vi "CHS-simulate-dashboard.vi"() -> ()   [LabVIEW 2019]
uses:
  Swerve_Drive_System/CHS_DRIVE_GLOBALS.vi
  Simulation/CHS_SIM_SIM_Globals.vi
  Trajectory Following/CHS_TRAJECTORY_GLOBALS.vi
  <vilib>/Rock Robotics/WPI/ThirdParty/JAS_Junk/TrajLib/Trajectory_Library.lvlib
  Vision_Interface/CHS_Vision_Globals.vi
  <vilib>/Rock Robotics/WPI/ThirdParty/ChoreoLib/ChoreoLib.lvlib
  <vilib>/Rock Robotics/WPI/ThirdParty/JAS_Junk/TrajLib/TypeDef/ROTATION2D.ctl
  <vilib>/Rock Robotics/WPI/ThirdParty/JAS_Junk/TrajLib/TypeDef/CHASSIS_SPEEDS.ctl
  <vilib>/Rock Robotics/WPI/ThirdParty/JAS_Junk/TrajLib/TypeDef/TRANSLATION2D.ctl
  <vilib>/Rock Robotics/WPI/ThirdParty/JAS_Junk/TrajLib/TypeDef/POSE2D.ctl
panel:
  in  "Tab Control":T1(tab)
  out "Mod Swerve in Deadband 2":bool
  out "Battery Voltage":dbl(graph)
  out "Swerve Motor Demands":T2(graph)
  out "Drive Motor Demands":T2(graph)
  out "Swerve Module Devices":T3(array[cluster])
  out "GyroReading_Degreees":dbl format="%15.3f"
  out "Encoder Distances":dbl[](array[numeric]) format="%17.2f"
  out "Encoder Velocities":dbl[](array[numeric]) format="%17.2f"
  out "Motor Demands":dbl[](array[numeric]) format="%17.2f"
  out "Battery Volts":dbl format="%16.2f"
  out "Mod Wheel \nSpeed Dmd":dbl[](array[numeric]) format="%17.3f"
  out "Swerve Drive Motor output":T4(graph)
  out "Swerve Drive Speed M/S":T5(graph)
  out "Swerve Drive Speed Error  M/S":T6(graph)
  out "Closed Loop Control":bool
  out "Orientation Angle Dmd_Rad":dbl format="%17.3f"
  out "Drv Chassis Adj Velocity DmD":T7 {"vOmega" format="%10.3f"; "vY" format="%10.3f"; "vX" format="%10.3f"}
  out "GyroHeading_Radians":dbl format="%17.2f"
  out "Orientation Angle Error_Rad":dbl format="%17.3f"
  out "Orientation Correct CO":dbl format="%17.3f"
  out "Swerve Chassis Speed":T7 {"vOmega" format="%10.3f"; "vY" format="%10.3f"; "vX" format="%10.3f"}
  out "Mod Swerve in Deadband":bool
  out "Mod Wheel Out":dbl[](array[numeric]) format="%17.3f"
  out "Mod Wheel \nSpeed M/S":dbl[](array[numeric]) format="%17.3f"
  out "Mod Wheel Speed Err":dbl[](array[numeric]) format="%17.3f"
  out "Opt Mod Wheel \nSpeed Dmd":dbl[](array[numeric]) format="%17.3f"
  out "Swerve Pos Dmd\nRadians":dbl[](array[numeric]) format="%17.3f"
  out "Optimized Swerve\nPos Dmd":dbl[](array[numeric]) format="%17.3f"
  out "Sweve Module Motor Output":T8(graph)
  out "Swerve Modue Position Radians":T5(graph)
  out "Swerve Module Position Error\nRadians":T9(graph)
  out "Closed Loop Control 2":bool
  out "Mod Swerve in Deadband 3":bool
  out "Mod Swerve Err  Radians":dbl[](array[numeric]) format="%17.3f"
  out "Mod Swerve Motor Out":dbl[](array[numeric]) format="%17.3f"
  out "Mod Pos Radians":dbl[](array[numeric]) format="%17.3f"
  out "Mod Swerve On Targ":bool[](array[boolean])
  out "Vision Pose":T10={"TRANSLATION"={"X"=0.0, "Y"=0.0}, "ROTATION"={"VALUE"=0.0, "COS"=1.0, "SIN"=0.0}} {"ROTATION"."SIN" format="%13.4f"; "ROTATION"."COS" format="%13.4f"; "ROTATION"."VALUE" format="%13.4f"; "TRANSLATION"."Y" format="%14.3f"; "TRANSLATION"."X" format="%14.3f"}
  out "Vision\nPose":bool
  out "Trajectory Status":T13(graph)
  out "Trajectory Execution \nClosed Loop":bool
  out "Mod Swerve in \nDeadband 3":bool
  out "Trajectory Error":T14(graph)
  out "Traj_OnTarget":bool
  out "Traj Heading Dmd Deg":dbl format="%17.2f"
  out "Traj Final Heading Dmd Deg":dbl format="%17.2f"
  out "Traj Sample Time Sec":dbl format="%17.2f"
  out "Traj Rot Vel FF Rad/Sec":dbl format="%17.2f"
  out "Relative Trajectory Pose":T10={"TRANSLATION"={"X"=0.0, "Y"=0.0}, "ROTATION"={"VALUE"=0.0, "COS"=1.0, "SIN"=0.0}} {"ROTATION"."SIN" format="%13.4f"; "ROTATION"."COS" format="%13.4f"; "ROTATION"."VALUE" format="%13.4f"; "TRANSLATION"."Y" format="%14.3f"; "TRANSLATION"."X" format="%14.3f"}
  out "Absolute Odometry \nPose":T10={"TRANSLATION"={"X"=0.0, "Y"=0.0}, "ROTATION"={"VALUE"=0.0, "COS"=1.0, "SIN"=0.0}} {"ROTATION"."SIN" format="%13.4f"; "ROTATION"."COS" format="%13.4f"; "ROTATION"."VALUE" format="%13.4f"; "TRANSLATION"."Y" format="%14.3f"; "TRANSLATION"."X" format="%14.3f"}
  out "Other ABS Odometry\nPose":T10={"TRANSLATION"={"X"=0.0, "Y"=0.0}, "ROTATION"={"VALUE"=0.0, "COS"=1.0, "SIN"=0.0}} {"ROTATION"."SIN" format="%13.4f"; "ROTATION"."COS" format="%13.4f"; "ROTATION"."VALUE" format="%13.4f"; "TRANSLATION"."Y" format="%14.3f"; "TRANSLATION"."X" format="%14.3f"}
  out "Absolue Trajectory":cluster{dbl[], dbl[]}(graph)
  out "Relative Trajectory":cluster{dbl[], dbl[]}(graph)
  # "SIMULATION"
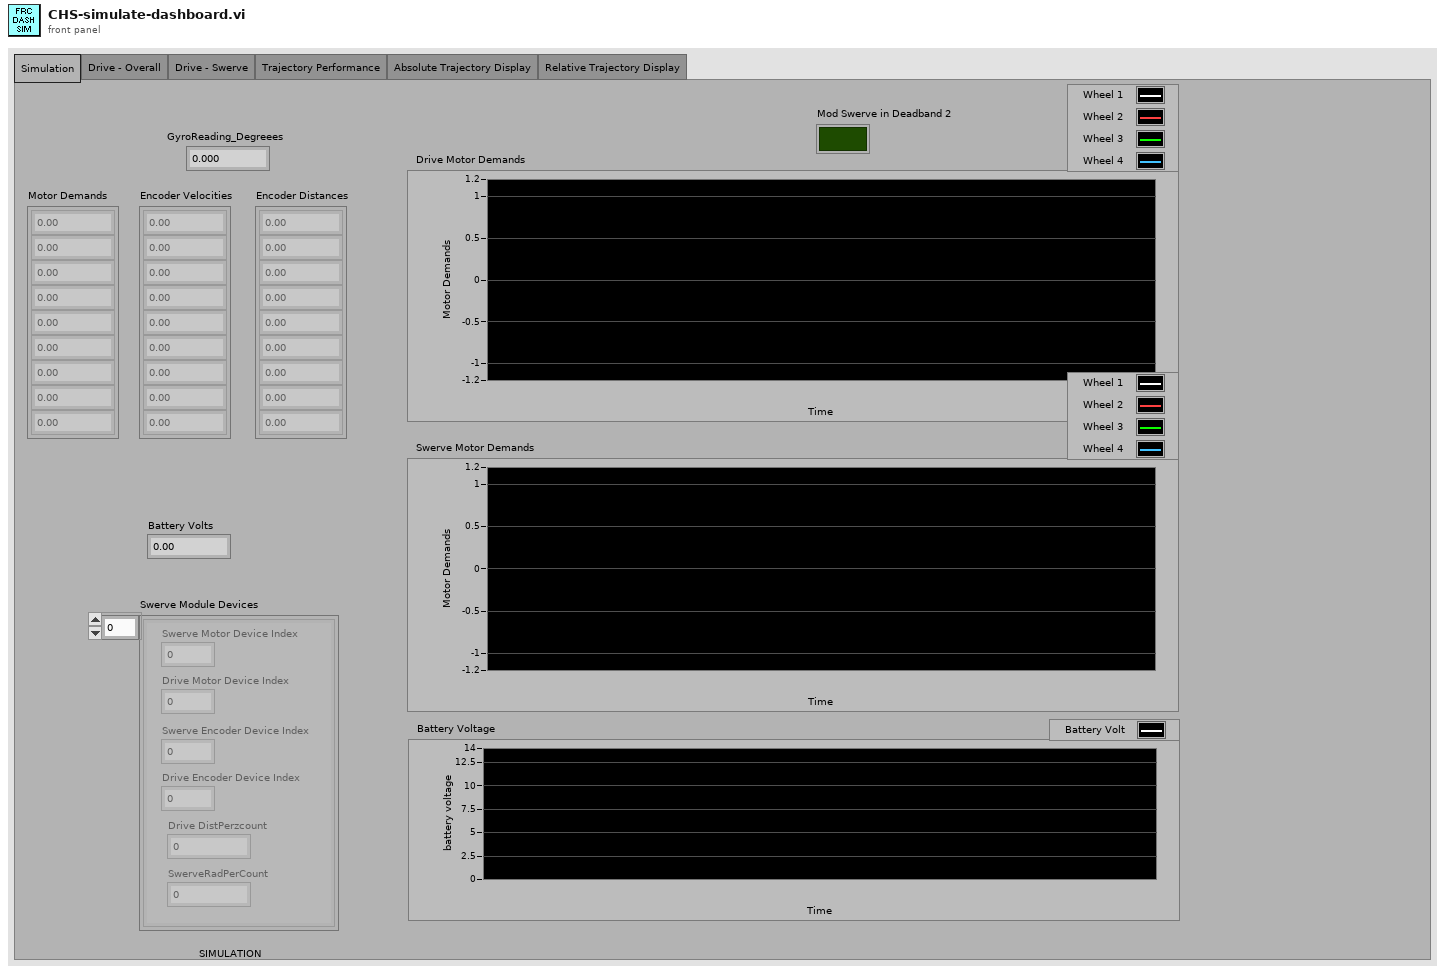
[diagram p1: front panel]
types:
  T1 = enum32{"Simulation", "Drive - Overall", "Drive - Swerve", "Trajectory Performance", "Absolute Trajectory Display", "Relative Trajectory Display"}
  T2 = cluster{"Motor Dmd":dbl, "Motor Dmd":dbl, "Motor Dmd":dbl, "Motor Dmd":dbl}
  T3 = cluster{"Swerve Motor Device Index":i32, "Drive Motor Device Index":i32, "Swerve Encoder Device Index":i32, "Drive Encoder Device Index":i32, "Drive DistPerzcount":dbl, "SwerveRadPerCount":dbl}[]
  T4 = cluster{"Mod Wheel Out[0]":dbl, "Mod Wheel Out[1]":dbl, "Mod Wheel Out[2]":dbl, "Mod Wheel Out[3]":dbl}
  T5 = cluster{"Angle RADIANS":dbl, "Angle RADIANS":dbl, "Angle RADIANS":dbl, "Distance M":dbl}
  T6 = cluster{"Mod Wheel Speed Err[0]":dbl, "Mod Wheel Speed Err[1]":dbl, "Mod Wheel Speed Err[2]":dbl, "Mod Wheel Speed Err[3]":dbl}
  T7 = typedef "Trajectory_Library.lvlib/CHASSIS_SPEEDS.ctl" = cluster{"vX":dbl, "vY":dbl, "vOmega":dbl}
  T8 = cluster{"Mod Swerve Out[0]":dbl, "Mod Swerve Out[1]":dbl, "Mod Swerve Out[2]":dbl, "Mod Swerve Out[3]":dbl}
  T9 = cluster{"Mod Swerve Err[0]":dbl, "Mod Swerve Err[1]":dbl, "Mod Swerve Err[2]":dbl, "Mod Swerve Err[3]":dbl}
  T10 = typedef "Trajectory_Library.lvlib/POSE2D.ctl" = cluster{"TRANSLATION":T11, "ROTATION":T12}
  T11 = typedef "Trajectory_Library.lvlib/TRANSLATION2D.ctl" = cluster{"X":dbl, "Y":dbl}
  T12 = typedef "Trajectory_Library.lvlib/ROTATION2D.ctl" = cluster{"VALUE":dbl, "COS":dbl, "SIN":dbl}
  T13 = cluster{dbl, dbl, dbl, "Traj_Sample_Time_Sec":dbl}
  T14 = cluster{"Traj X Err":dbl, "Traj Y Err":dbl, "Traj Heading Err":dbl}
  T15 = cluster{"Traj X Err_FT":dbl, "Traj Y Err_FT":dbl, "Traj Heading Err_DEG":dbl}
  T16 = typedef "Trajectory_Library.lvlib/SWERVE_DRIVE_MODULE_POSITION.ctl" = cluster{"Distance":dbl, "Angle":T12, "P":bool}
  T17 = typedef "ChoreoLib.lvlib/ChoreoTrajectory.ctl" = T18[]
  T18 = typedef "ChoreoLib.lvlib/ChoreoTrajectoryState.ctl" = cluster{"timestamp":dbl, "x":dbl, "y":dbl, "heading":dbl, "velocityX":dbl, "velocityY":dbl, "angularVelocity":dbl}
  T19 = typedef "Trajectory_Library.lvlib/SWERVE_DRIVE_MODULE_STATE.ctl" = cluster{"Speed":dbl, "Angle":T12}
  T20 = cluster{"Angle RADIANS":dbl, "Angle RADIANS":dbl, "Angle RADIANS":dbl, "Angle RADIANS":dbl}
  T21 = cluster{"Speed M/S":dbl, "Speed M/S":dbl, "Speed M/S":dbl, "Speed M/S":dbl}
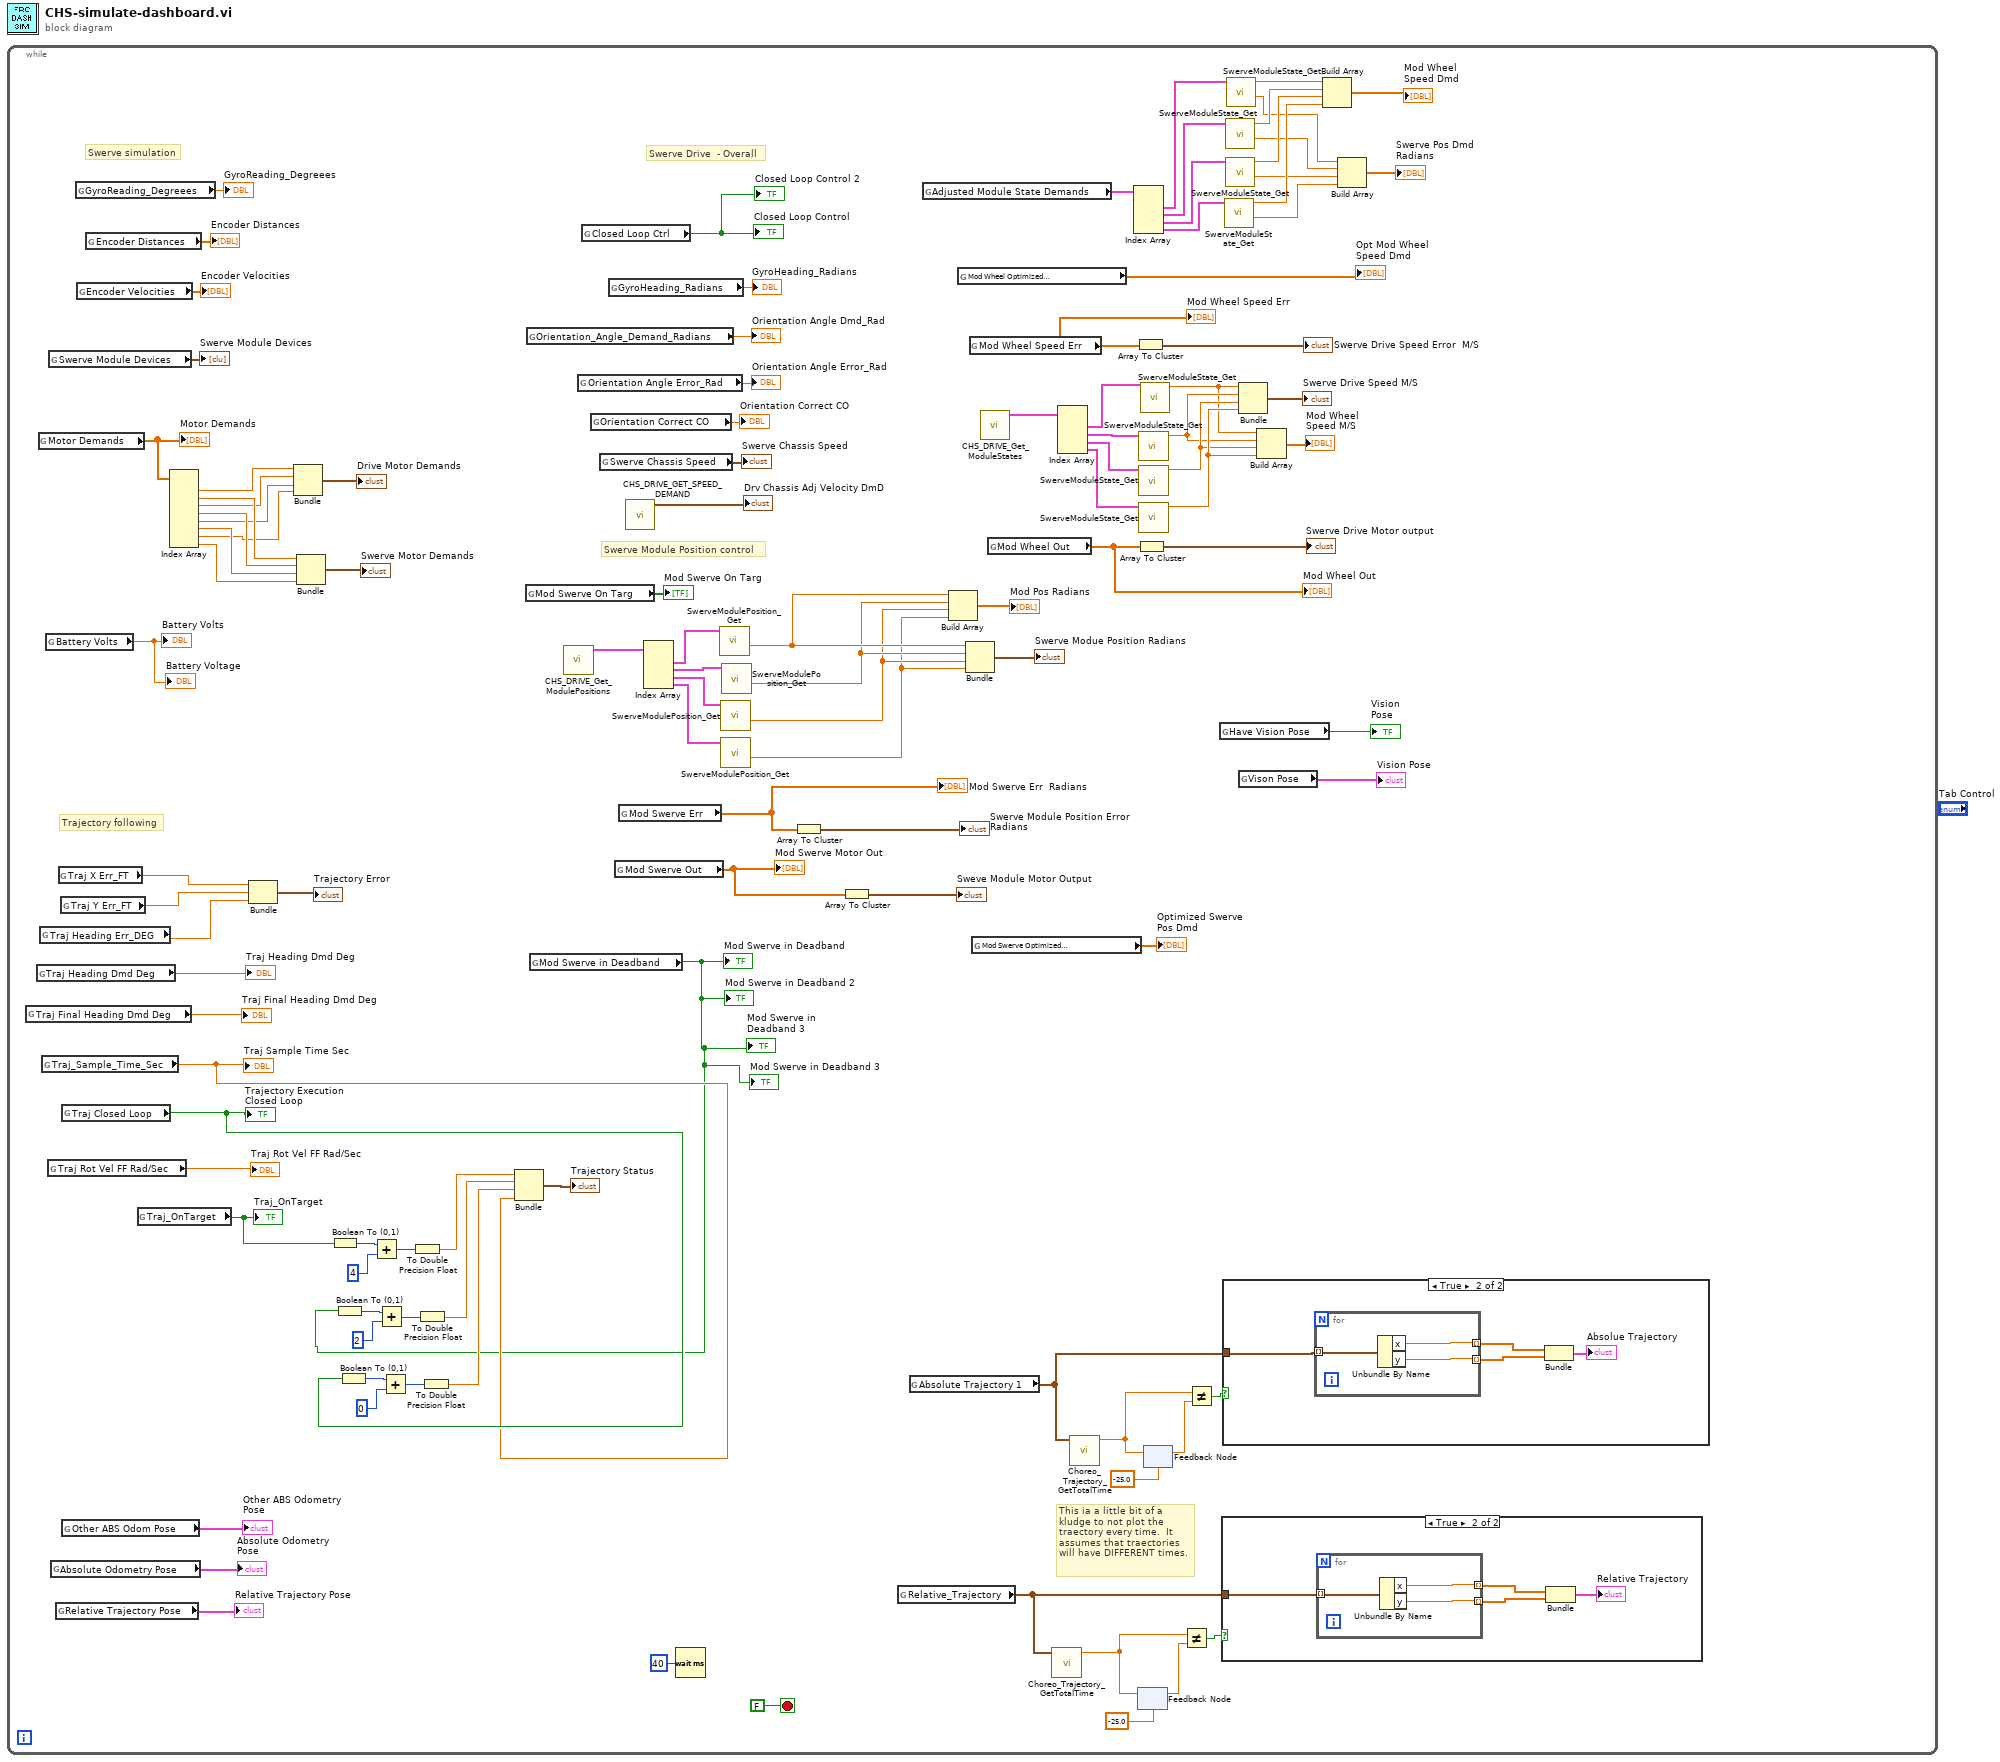
[diagram p0: block diagram]
diagram:
  n1 = while {
    stop <- FALSE stop-if-true
    # "This ia a little bit of a \nkludge to not plot the\ntraectory every time.  It \nassumes that traectories\nwill have DIFFERENT times."
    # "Swerve Module Position control"
    # "Trajectory following"
    # "Swerve simulation"
    # "Swerve Drive  - Overall"
    n2 = global read "CHS_TRAJECTORY_GLOBALS.vi" "Traj Final Heading Dmd Deg"() -> (→"Traj Final Heading Dmd Deg":dbl)
    n3 = global read "CHS_TRAJECTORY_GLOBALS.vi" "Traj Heading Dmd Deg"() -> (→"Traj Heading Dmd Deg":dbl)
    n4 = global read "CHS_SIM_SIM_Globals.vi" "Motor Demands"() -> (w99:dbl[])
    "Motor Demands" <- w99
    n5 = global read "CHS_TRAJECTORY_GLOBALS.vi" "Traj Heading Err_DEG"() -> (w86:dbl)
    n6 = global read "CHS_TRAJECTORY_GLOBALS.vi" "Traj_Sample_Time_Sec"() -> (w67:dbl)
    "Traj Sample Time Sec" <- w67
    n7 = global read "CHS_SIM_SIM_Globals.vi" "Battery Volts"() -> (→"Battery Volts" →"Battery Voltage":dbl)
    n8 = global read "CHS_TRAJECTORY_GLOBALS.vi" "Traj Rot Vel FF Rad/Sec"() -> (→"Traj Rot Vel FF Rad/Sec":dbl)
    n9 = global read "CHS_SIM_SIM_Globals.vi" "Swerve Module Devices"() -> (→"Swerve Module Devices":T3)
    n10 = global read "CHS_TRAJECTORY_GLOBALS.vi" "Absolute Odometry Pose"() -> (→"Absolute Odometry \nPose":T10)
    n11 = global read "CHS_TRAJECTORY_GLOBALS.vi" "Relative Trajectory Pose"() -> (→"Relative Trajectory Pose":T10)
    n12 = global read "CHS_TRAJECTORY_GLOBALS.vi" "Traj X Err_FT"() -> (w88:dbl)
    n13 = global read "CHS_TRAJECTORY_GLOBALS.vi" "Traj Y Err_FT"() -> (w87:dbl)
    n14 = global read "CHS_TRAJECTORY_GLOBALS.vi" "Traj Closed Loop"() -> (w69:bool)
    "Trajectory Execution \nClosed Loop" <- w69
    n15 = global read "CHS_TRAJECTORY_GLOBALS.vi" "Other ABS Odom Pose"() -> (→"Other ABS Odometry\nPose":T10)
    n16 = global read "CHS_SIM_SIM_Globals.vi" "GyroReading_Degreees"() -> (→"GyroReading_Degreees":dbl)
    n17 = global read "CHS_SIM_SIM_Globals.vi" "Encoder Velocities"() -> (→"Encoder Velocities":dbl[])
    n18 = global read "CHS_SIM_SIM_Globals.vi" "Encoder Distances"() -> (→"Encoder Distances":dbl[])
    n19 = global read "CHS_TRAJECTORY_GLOBALS.vi" "Traj_OnTarget"() -> (w81:bool)
    "Traj_OnTarget" <- w81
    n20 = Index Array(array=w99) -> (element #1=w98:dbl, element #2=w97:dbl, element #3=w96:dbl, element #4=w95:dbl, element #5=w94:dbl, element #6=w93:dbl, element #7=w92:dbl, element #8=w91:dbl)  [unwired: 8 in]
    n21 = Bundle("Traj X Err_FT"=w88, "Traj Y Err_FT"=w87, "Traj Heading Err_DEG"=w86) -> (→"Trajectory Error":T15)  [unwired: 1 in]
    n22 = Bundle("Motor Dmd"=w98, "Motor Dmd"=w96, "Motor Dmd"=w94, "Motor Dmd"=w92) -> (→"Drive Motor Demands":T2)  [unwired: 1 in]
    n23 = Bundle("Motor Dmd"=w97, "Motor Dmd"=w95, "Motor Dmd"=w93, "Motor Dmd"=w91) -> (→"Swerve Motor Demands":T2)  [unwired: 1 in]
    n24 = Boolean To (0,1)(Boolean=w81) -> (0, 1=w79:i16)
    n25 = Boolean To (0,1)(Boolean=w69) -> (0, 1=w72:i16)
    n26 = Add(x=w79, y=i16 4) -> (x+y=w78:i16)
    n27 = Add(x=w72, y=i16 0) -> (x+y=w71:i16)
    n28 = To Double Precision Float(number=w78) -> (double precision float=w80:dbl)
    n29 = To Double Precision Float(number=w71) -> (double precision float=w68:dbl)
    n30 = global read "CHS_DRIVE_GLOBALS.vi" "Mod Swerve On Targ"() -> (→"Mod Swerve On Targ":bool[])
    n31 = global read "CHS_DRIVE_GLOBALS.vi" "Orientation_Angle_Demand_Radians"() -> (→"Orientation Angle Dmd_Rad":dbl)
    n32 = global read "CHS_DRIVE_GLOBALS.vi" "Mod Swerve in Deadband"() -> (w53:bool)
    "Mod Swerve in Deadband" <- w53
    "Mod Swerve in Deadband 2" <- w53
    "Mod Swerve in \nDeadband 3" <- w53
    "Mod Swerve in Deadband 3" <- w53
    n33 = Boolean To (0,1)(Boolean=w53) -> (0, 1=w76:i16)
    n34 = Add(x=w76, y=i16 2) -> (x+y=w75:i16)
    n35 = To Double Precision Float(number=w75) -> (double precision float=w73:dbl)
    n36 = Bundle(w80, w73, w68, "Traj_Sample_Time_Sec"=w67) -> (→"Trajectory Status":T13)  [unwired: 1 in]
    n37 = call "CHS_DRIVE_Get_ModulePositions.vi"() -> ("Swerve Module Positions"=w62:T16[])  [unwired: 11 in]
    n38 = global read "CHS_DRIVE_GLOBALS.vi" "Orientation Angle Error_Rad"() -> (→"Orientation Angle Error_Rad":dbl)
    n39 = global read "CHS_DRIVE_GLOBALS.vi" "Closed Loop Ctrl"() -> (→"Closed Loop Control" →"Closed Loop Control 2":bool)
    n40 = global read "CHS_DRIVE_GLOBALS.vi" "Orientation Correct CO"() -> (→"Orientation Correct CO":dbl)
    n41 = global read "CHS_DRIVE_GLOBALS.vi" "Swerve Chassis Speed"() -> (→"Swerve Chassis Speed":T7)
    n42 = global read "CHS_DRIVE_GLOBALS.vi" "GyroHeading_Radians"() -> (→"GyroHeading_Radians":dbl)
    n43 = global read "CHS_DRIVE_GLOBALS.vi" "Mod Swerve Out"() -> (w41:dbl[])
    "Mod Swerve Motor Out" <- w41
    n44 = global read "CHS_DRIVE_GLOBALS.vi" "Mod Swerve Err"() -> (w57:dbl[])
    "Mod Swerve Err  Radians" <- w57
    n45 = call "CHS_DRIVE_GET_SPEED_DEMAND.vi"() -> ("Drv Chassis Velocity DmD"=→"Drv Chassis Adj Velocity DmD":T7)  [unwired: 11 in]
    n46 = Index Array(array=w62) -> (element #1=w61:T16, element #2=w60:T16, element #3=w59:T16, element #4=w58:T16)  [unwired: 4 in]
    n47 = Wait (ms)(milliseconds to wait=u32 40) -> ()  [unwired: 1 out]
    n48 = call <vilib>:"SwerveModulePosition_Get.vi"("Swerve Module Position"=w61) -> ("Angle RADIANS"=w40:dbl)  [unwired: 8 in, 2 out]
    n49 = call <vilib>:"SwerveModulePosition_Get.vi"("Swerve Module Position"=w59) -> ("Angle RADIANS"=w38:dbl)  [unwired: 8 in, 2 out]
    n50 = call <vilib>:"SwerveModulePosition_Get.vi"("Swerve Module Position"=w58) -> ("Angle RADIANS"=w37:dbl)  [unwired: 8 in, 2 out]
    n51 = call <vilib>:"SwerveModulePosition_Get.vi"("Swerve Module Position"=w60) -> ("Angle RADIANS"=w39:dbl)  [unwired: 8 in, 2 out]
    n52 = Array To Cluster(array=w57) -> (cluster=→"Swerve Module Position Error\nRadians":T9)
    n53 = Array To Cluster(array=w41) -> (cluster=→"Sweve Module Motor Output":T8)
    n54 = global read "CHS_TRAJECTORY_GLOBALS.vi" "Relative_Trajectory"() -> (w2:T17)
    n55 = global read "CHS_TRAJECTORY_GLOBALS.vi" "Absolute Trajectory 1"() -> (w4:T17)
    n56 = global read "CHS_DRIVE_GLOBALS.vi" "Adjusted Module State Demands"() -> (w30:T19[])
    n57 = Build Array(w40, w39, w38, w37) -> (→"Mod Pos Radians":dbl[])
    n58 = global read "CHS_DRIVE_GLOBALS.vi" "Mod Wheel Optimized \nDmd"() -> (→"Opt Mod Wheel \nSpeed Dmd":dbl[])
    n59 = Bundle("Angle RADIANS"=w40, "Angle RADIANS"=w39, "Angle RADIANS"=w38, "Angle RADIANS"=w37) -> (→"Swerve Modue Position Radians":T20)  [unwired: 1 in]
    n60 = global read "CHS_DRIVE_GLOBALS.vi" "Mod Wheel Speed Err"() -> (w56:dbl[])
    "Mod Wheel Speed Err" <- w56
    n61 = global read "CHS_DRIVE_GLOBALS.vi" "Mod Swerve Optimized\nDmd"() -> (→"Optimized Swerve\nPos Dmd":dbl[])
    n62 = call "CHS_DRIVE_Get_ModuleStates.vi"() -> ("Swerve Module States"=w50:T19[])  [unwired: 11 in]
    n63 = global read "CHS_DRIVE_GLOBALS.vi" "Mod Wheel Out"() -> (w44:dbl[])
    "Mod Wheel Out" <- w44
    n64 = call <vilib>:"Choreo_Trajectory_GetTotalTime.vi"("ChoreoTrajectory"=w2) -> ("timestamp"=w1:dbl)  [unwired: 10 in]
    n65 = Index Array(array=w50) -> (element #1=w48:T19, element #2=w49:T19, element #3=w47:T19, element #4=w46:T19)  [unwired: 4 in]
    n66 = call <vilib>:"Choreo_Trajectory_GetTotalTime.vi"("ChoreoTrajectory"=w4) -> ("timestamp"=w3:dbl)  [unwired: 10 in]
    n67 = Index Array(array=w30) -> (element #1=w29:T19, element #2=w28:T19, element #3=w27:T19, element #4=w26:T19)  [unwired: 4 in]
    n68 = Array To Cluster(array=w56) -> (cluster=→"Swerve Drive Speed Error  M/S":T6)
    n69 = Array To Cluster(array=w44) -> (cluster=→"Swerve Drive Motor output":T4)
    n70 = feedback #1(-25.0 ("TotalTime_Sec")) -> (w6:dbl)
    n71 = feedback-in #1(w1) -> ()
    n72 = call <vilib>:"SwerveModuleState_Get.vi"("Desired State"=w49) -> ("Speed M/S"=w32:dbl)  [unwired: 9 in, 1 out]
    n73 = call <vilib>:"SwerveModuleState_Get.vi"("Desired State"=w47) -> ("Speed M/S"=w33:dbl)  [unwired: 9 in, 1 out]
    n74 = call <vilib>:"SwerveModuleState_Get.vi"("Desired State"=w46) -> ("Speed M/S"=w34:dbl)  [unwired: 9 in, 1 out]
    n75 = call <vilib>:"SwerveModuleState_Get.vi"("Desired State"=w48) -> ("Speed M/S"=w31:dbl)  [unwired: 9 in, 1 out]
    n76 = feedback #2(-25.0 ("TotalTime_Sec")) -> (w9:dbl)
    n77 = feedback-in #2(w3) -> ()
    n78 = Not Equal?(x=w1, y=w6) -> (x != y?=w5:bool)
    n79 = Not Equal?(x=w3, y=w9) -> (x != y?=w8:bool)
    n80 = global read "CHS_Vision_Globals.vi" "Have Vision Pose"() -> (→"Vision\nPose":bool)
    n81 = case shown="True" w5 {
      tunnel: w2 -> [_ w113]
      frame False {
      }
      frame True {
        n82 = for {
          tunnel: [w119] -> w115 mode=indexing
          tunnel: [w118] -> w116 mode=indexing
          tunnel: w113 -> [w117] mode=indexing
          n83 = Unbundle By Name(w117) -> ("x"=w119:dbl, "y"=w118:dbl)
        }
        n84 = Bundle(w115, w116) -> (→"Relative Trajectory":cluster{dbl[], dbl[]})  [unwired: 1 in]
      }
    }
    n85 = case shown="True" w8 {
      tunnel: w4 -> [_ w120]
      frame False {
      }
      frame True {
        n86 = for {
          tunnel: [w126] -> w122 mode=indexing
          tunnel: [w125] -> w123 mode=indexing
          tunnel: w120 -> [w124] mode=indexing
          n87 = Unbundle By Name(w124) -> ("x"=w126:dbl, "y"=w125:dbl)
        }
        n88 = Bundle(w122, w123) -> (→"Absolue Trajectory":cluster{dbl[], dbl[]})  [unwired: 1 in]
      }
    }
    n89 = call <vilib>:"SwerveModuleState_Get.vi"("Desired State"=w26) -> ("Angle RADIANS"=w16:dbl, "Speed M/S"=w22:dbl)  [unwired: 9 in]
    n90 = call <vilib>:"SwerveModuleState_Get.vi"("Desired State"=w28) -> ("Angle RADIANS"=w18:dbl, "Speed M/S"=w24:dbl)  [unwired: 9 in]
    n91 = call <vilib>:"SwerveModuleState_Get.vi"("Desired State"=w27) -> ("Angle RADIANS"=w17:dbl, "Speed M/S"=w23:dbl)  [unwired: 9 in]
    n92 = call <vilib>:"SwerveModuleState_Get.vi"("Desired State"=w29) -> ("Angle RADIANS"=w19:dbl, "Speed M/S"=w25:dbl)  [unwired: 9 in]
    n93 = Bundle("Speed M/S"=w31, "Speed M/S"=w32, "Speed M/S"=w33, "Speed M/S"=w34) -> (→"Swerve Drive Speed M/S":T21)  [unwired: 1 in]
    n94 = global read "CHS_Vision_Globals.vi" "Vison Pose"() -> (→"Vision Pose":T10)
    n95 = Build Array(w31, w32, w33, w34) -> (→"Mod Wheel \nSpeed M/S":dbl[])
    n96 = Build Array(w25, w24, w23, w22) -> (→"Mod Wheel \nSpeed Dmd":dbl[])
    n97 = Build Array(w19, w18, w17, w16) -> (→"Swerve Pos Dmd\nRadians":dbl[])
  }
